vi "PlotPosition.vi"() -> ()   [LabVIEW 2010]
panel:
  in  "Motor GPIB":u8=6
  out "XY Graph":cluster{"Y":dbl[], "Y":dbl[]}[](graph)
  out "x":i32
  out "y":i32
  out "Loop count":i32
  in  "stop":bool
  out "y-disp":i32[](array[numeric])
  out "x-disp":i32[](array[numeric])
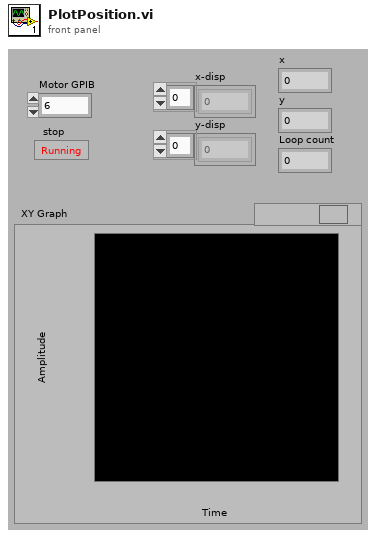
[diagram p1: front panel]
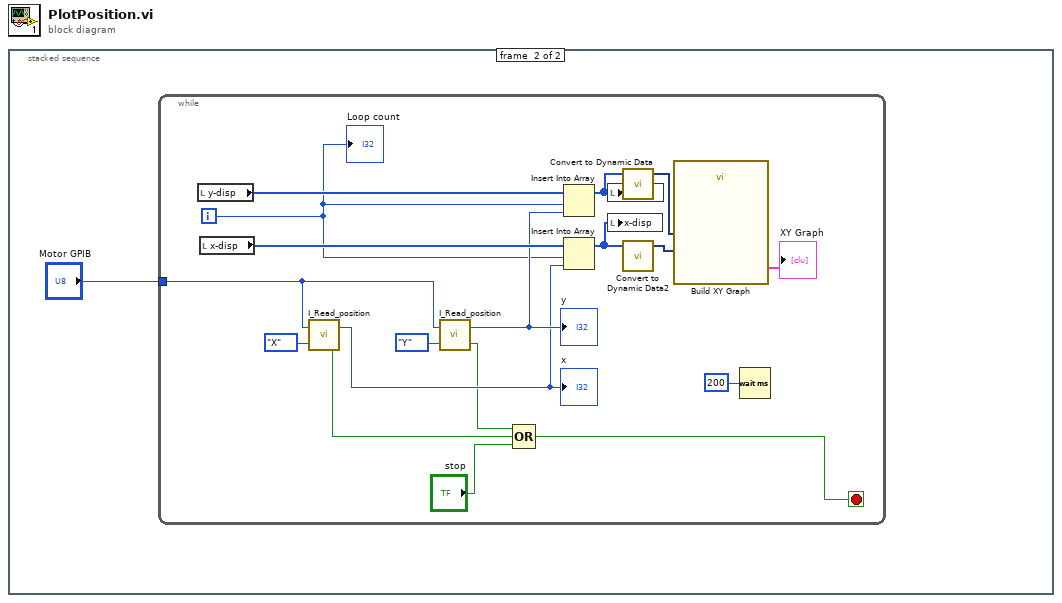
[diagram p0: block diagram]
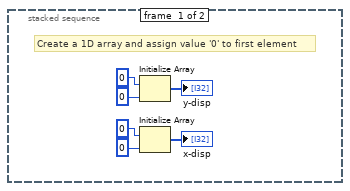
[diagram p2: hidden frame]
diagram:
  n1 = stacked-sequence {
    frame #0 {
      # "Create a 1D array and assign value '0' to first element"
      n2 = Initialize Array(0 ("element"), 0 ("dimension size")) -> (→"y-disp":i32[])
      n3 = Initialize Array(0 ("element"), 0 ("element")) -> (→"x-disp":i32[])
    }
    frame #1 {
      n4 = while {
        tunnel: "Motor GPIB" -> [w10]
        i -> [w15]
        stop <- w11 stop-if-true
        n5 = local read "y-disp"() -> (w24:i32[])
        n6 = local read "x-disp"() -> (w25:i32[])
        n7 = call "I_Read_position.vi"("Axis"=enum16{"X", "Y", "Z", "U", "V", "W"}."X", "Motor GPIB"=w10) -> ("Error?"=w13:bool, "Position"=w19:i32)
        "x" <- w19
        n8 = call "I_Read_position.vi"("Axis"=enum16{"X", "Y", "Z", "U", "V", "W"}."Y", "Motor GPIB"=w10) -> ("Error?"=w14:bool, "Position"=w20:i32)
        "y" <- w20
        n9 = Compound Arithmetic op=OR(w14, w13, "stop") -> (w11:bool)
        n10 = Insert Into Array(array=w24, index=w15, new element=w20) -> (w18:i32[])
        n11 = Insert Into Array(array=w25, index=w15, new element=w19) -> (w17:i32[])
        n12 = local write "y-disp"(w18) -> ()
        n13 = local write "x-disp"(w17) -> ()
        n14 = call "Convert to Dynamic Data"("Array"=w18) -> ("Dynamic Data Type"=w23:dynamicdata)  [unwired: 3 in]
        n15 = call "Convert to Dynamic Data2"("Array"=w17) -> ("Dynamic Data Type"=w22:dynamicdata)  [unwired: 3 in]
        n16 = call "Build XY Graph"("Y Input"=w22, "X Input"=w23) -> ("XY Graph"=→"XY Graph":cluster{"Y":dbl[], "Y":dbl[]}[])  [unwired: 3 in, 6 out]
        n17 = Wait (ms)(milliseconds to wait=u32 200) -> ()  [unwired: 1 out]
        "Loop count" <- w15
      }
    }
  }
